vi "Upd State.vi"(8 "error in (no error)":errorcluster, 10 "Upd State":bool, 11 "Mech Pump in":refnum<class "Mech Pump.lvclass">) -> (0 "error out":errorcluster, 3 "Mech Pump out":refnum<class "Mech Pump.lvclass">)   [LabVIEW 2021, in "Mech Pump.lvlib" / "Mech Pump.lvclass"]
uses:
  Mech Pump.lvclass
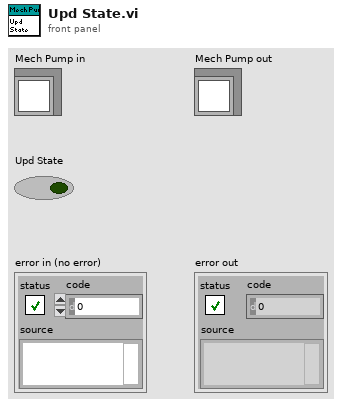
[diagram p1: front panel]
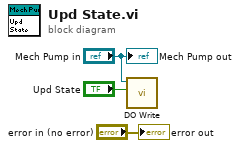
[diagram p0: block diagram]
diagram:
  n1 = call "DO Write.vi"("Digital Output"="Upd State", "Mech Pump in"="Mech Pump in") -> ()  [unwired: 9 in, 1 out]
  "error out" <- "error in (no error)"
  "Mech Pump out" <- "Mech Pump in"
